vi "TDC_DAQV29_Paralled_muon.vi"(7 "address":string[](array[string])=["192.168.10.20"], 8 "error in (no error)":errorcluster, 9 "stop":bool, 10 "save data":bool=TRUE, 11 "SMA mode":bool) -> (0 "error out 3":errorcluster, 2 "csv path":path=path "D:/tdc/2017/data/test_20250311_101020.csv", 3 "rate":dbl=1.0823196338413628)   [LabVIEW 2017]
uses:
  gloabal.vi
  <vilib>/Utility/file.llb/Write Delimited Spreadsheet (DBL).vi
  <vilib>/Utility/file.llb/Write Delimited Spreadsheet (I64).vi
panel:
  out "pmt trigger rate":u32[](array[numeric])=[0, 35, 51, 19, 33, 19, 2704, 0, 64, 55, 26, 21, 70, 31, 43, 33, 76, 251, 28, 323, 16, 59, 106, 98, 0, 13, 2, 0, 53, 3, 0, 21, 65, 24, 240, 3, 89, 7, 48, 4, 0, 1, 60, 40, 0, 96, 100, 5, 11, 3, 0, 0, 0, 0, 0, 0, 0, 0, 0, 0, 0, 0, 0, 0]
  out "trigger rate":u64 format="%x"
  out "event":u32[](array[numeric])=[0, 0, 169, 166, 205, 191, 115, 111, 155, 143, 118, 110, 11836, 10970, 0, 0, 225, 211, 261, 248, 128, 116, 109, 106, 298, 278, 156, 146, 231, 218, 149, 126, 334, 315, 1087, 1060, 180, 172, 1669, 1652, 100, 96, 371, 351, 355, 349, 389, 370, 1, 1, 62, 58, 6, 6, 0, 0, 259, 253, 9, 8, 0, 0, 106, 100, 234, 213, 109, 106, 1110, 1086, 10, 9, 391, 374, 24, 24, 280, 267, 12, 12, 0, 0, 2, 2, 293, 271, 143, 136, 3, 3, 279, 187, 492, 458, 14, 13, 37, 35, 9, 8, 0, 0, 0, 0, 0, 0, 0, 0, 0, 0, 0, 0, 0, 0, 0, 0, 0, 0, 0, 0, 0, 0, 0, 0, 0, 0, 0, 0]
  in  "calib_file":path=path "D:/tdc/2017/data/test_20250311_110721_codeDensity.csv" caption="文件路径 （空时为对话框）"
  in  "use_calib_file":bool=TRUE
  out "cal 3":u32[](graph)=[0, 0, 0, 0, 0, 0, 0, 0, 0, 0, 0, 0, 0, 0, 0, 0, 0, 0, 0, 0, 0, 0, 0, 0, 0, 0, 0, 0, 0, 0, 0, 0, 0, 0, 0, 0, 0, 0, 0, 0, 0, 0, 0, 0, 0, 0, 0, 0, 0, 0, 0, 0, 0, 0, 0, 0, 0, 0, 0, 0, 0, 0, 0, 0, 0, 0, 0, 0, 0, 0, 0, 0, 0, 0, 0, 0, 0, 0, 0, 0, 0, 0, 0, 0, 0, 0, 0, 0, 0, 0, 0, 0, 0, 0, 0, 0, 0, 0, 0, 0, 0, 0, 0, 0, 0, 0, 0, 0, 0, 0, 0, 0, 0, 0, 0, 0, 0, 0, 0, 0, 0, 0, 0, 0, 0, 0, 0, 0, 0, 0, 0, 0, 0, 0, 0, 0, 0, 0, 0, 0, 0, 0, 0, 0, 0, 0, 0, 0, 0, 0, 0, 0, 0, 0, 0, 0, 0, 0, 0, 0, 0, 0, 0, 0, 0, 15, 3, 1, 14, 3, 31, 20, 16, 6, 1, 18, 12, 4, 29, 10, 8, 29, 2, 14, 4, 25, 7, 24, 4, 0, 1, 5, 8, 18, 22, 0, 4, 5, 0, 12, 9, 9, 20, 21, 4, 10, 13, 5, 21, 13, 14, 2, 6, 13, 1, 3, 5, 10, 20, 2, 3, 4, 3, 4, 2, 20, 13, 2, 5, 1, 3, 12, 4, 1, 14, 7, 5, 4, 1, 10, 2, 21, 14, 2, 5, 10, 4, 0, 11, 19, 6, 4, 1, 37, 1, 4, 2, 1, 10, 13, 4, 8, 10, 6, 9, 2, 0, 6, 8, 12, 3, 21, 5, 7, 8, 2, 3, 7, 17, 6, 5, 6, 4, 6, 0, 2, 1, 3, 10, 33, 7, 2, 6, 3, 7, 3, 2, 0, 12, 10, 11, 13, 13, 7, 3, 9, 6, 16, 0, 13, 5, 6, 3, 0, 5, 5, 7, 1, 10, 7, 13, 14, 5, 1, 12, 7, 1, 10, 2, 1, 14, 18, 13, 11, 4, 6, 9, 22, 11, 9, 2, 2, 8, 14, 4, 4, 6, 12, 13, 3, 9, 5, 5, 1, 5, 11, 18, 3, 0, 5, 4, 6, 7, 6, 1, 13, 5, 1, 2, 2, 1, 4, 12, 7, 3, 2, 3, 9, 11, 1, 20, 3, 4, 5, 5, 3, 5, 8, 5, 3, 26, 14, 6, 1, 3, 12, 12, 4, 23, 10, 3, 4, 4, 10, 3, 5, 4, 2, 14, 5, 15, 20, 1, 5, 1, 20, 6, 1, 3, 13, 21, 12, 7, 4, 1, 5, 30, 11, 2, 4, 0, 12, 7, 10, 3, 2, 25, 6, 1, 3, 6, 3, 8, 37, 4, 6, 2, 2, 4, 3, 5, 6, 13, 6, 9, 22, 1, 3, 7, 7, 4, 8, 33, 2, 1, 15, 3, 8, 23, 21, 2, 2, 27, 13, 3, 5, 10, 4, 18, 5, 5, 8, 0, 1, 8, 12, 4, 3, 0, 4, 8, 4, 7, 4, 2, 11, 13, 3, 0, 7, 5, 3, 4, 8, 4, 20, 2, 13, 4, 8, 6, 17, 4, 2, 1, 15, 2, 15, 5, 19, 0, 4, 15, 4, 16, 11, 1, 16, 4, 6, 6, 5, 7, 3, 9, 15, 3, 6, 3, 13, 5, 7, 3, 27, 2, 0, 21, 1, 4, 1, 4, 5, 3, 10, 7, 3, 6, 4, 18, 21, 7, 6, 7, 7, 12, 6, 9, 8, 11, 12, 13, 2, 2, 5, 4, 7, 52, 3, 5, 8, 7, 10, 4, 4, 6, 5, 18, 0, 3, 6, 1, 9, 5, 19, 13, 24, 12, 4, 4, 15, 6, 41, 3, 8, 5, 17, 26, 8, 7, 20, 2, 5, 12, 10, 10, 12, 9, 17, 6, 3, 1, 5, 3, 7, 8, 4, 10, 5, 10, 7, 1, 2, 14, 7, 25, 3, 0, 0, 0, 5, 21, 8, 14, 4, 10, 2, 3, 2, 4, 8, 12, 3, 6, 8, 3, 4, 3, 20, 5, 6, 7, 8, 11, 2, 8, 6, 5, 15, 17, 10, 10, 3, 3, 9, 18, 7, 7, 3, 5, 5, 5, 2, 2, 2, 4, 1, 0, 42, 3, 14, 4, 3, 5, 2, 7, 4, 2, 7, 5, 22, 4, 3, 17, 3, 5, 8, 19, 7, 5, 0, 3, 4, 10, 1, 8, 2, 2, 13, 23, 4, 9, 5, 0, 0, 0, 27, 2, 16, 11, 15, 3, 0, 18, 2, 8, 29, 19, 6, 7, 2, 6, 12, 1, 13, 2, 7, 5, 11, 8, 5, 6, 6, 19, 2, 4, 0, 7, 22, 13, 3, 7, 3, 8, 11, 0, 3, 26, 6, 5, 5, 6, 4, 10, 17, 16, 4, 3, 4, 3, 4, 21, 8, 10, 10, 7, 0, 9, 9, 2, 10, 10, 2, 9, 9, 4, 14, 5, 5, 4, 18, 6, 3, 0, 4, 1, 20, 2, 33, 4, 1, 2, 1, 20, 6, 3, 11, 10, 2, 1, 13, 9, 6, 1, 0, 0, 0, 0, 0, 0, 0, 0, 0, 0, 0, 0, 0, 0, 0, 0, 0, 0, 0, 0, 0, 0, 0, 0, 0, 0, 0, 0, 0, 0, 0, 0, 0, 0, 0, 0, 0, 0, 0, 0, 0, 0, 0, 0, 0, 0, 0, 0, 0, 0, 0, 0, 0, 0, 0, 0, 0, 0, 0, 0, 0, 0, 0, 0, 0, 0, 0, 0, 0, 0, 0, 0, 0, 0, 0, 0, 0, 0, 0, 0, 0, 0, 0, 0, 0, 0, 0, 0, 0, 0, 0, 0, 0, 0, 0, 0, 0, 0, 0, 0, 0, 0, 0, 0, 0, 0, 0, 0, 0, 0, 0, 0, 0, 0, 0, 0, 0, 0, 0, 0, 0, 0, 0, 0, 0, 0, 0, 0, 0, 0, 0, 0, 0, 0, 0, 0, 0, 0, 0, 0, 0, 0, 0, 0, 0, 0, 0, 0, 0, 0, 0, 0, 0, 0, 0, 0, 0, 0, 0, 0, 0, 0, 0, 0, 0, 0, 0, 0, 0, 0, 0, 0, 0, 0, 0, 0, 0, 0, 0, 0, 0, 0, 0, 0, 0, 0, 0, 0, 0, 0, 0, 0, 0, 0, 0, 0, 0, 0, 0, 0, 0, 0, 0, 0, 0, 0, 0, 0, 0, 0, 0, 0, 0, 0, 0, 0, 0, 0, 0, 0, 0, 0, 0, 0, 0, 0, 0, 0, 0, 0, 0, 0, 0, 0, 0, 0, 0, 0, 0, 0, 0, 0, 0, 0, 0, 0, 0, 0, 0, 0, 0, 0, 0, 0, 0, 0, 0, 0, 0, 0, 0, 0, 0, 0, 0, 0, 0, 0, 0, 0, 0, 0, 0, 0, 0, 0, 0, 0, 0, 0, 0, 0, 0, 0, 0, 0, 0, 0, 0, 0, 0, 0, 0, 0, 0, 0, 0, 0, 0, 0, 0, 0, 0, 0, 0, 0, 0, 0, 0, 0, 0, 0, 0, 0, 0, 0, 0, 0, 0, 0, 0, 0, 0, 0, 0, 0, 0, 0, 0, 0, 0, 0, 0, 0, 0, 0, 0, 0, 0, 0, 0, 0, 0, 0, 0, 0, 0, 0, 0, 0, 0, 0, 0, 0, 0, 0, 0, 0, 0, 0, 0, 0, 0, 0, 0, 0, 0, 0, 0, 0, 0, 0, 0, 0, 0, 0, 0, 0, 0, 0, 0, 0, 0, 0, 0, 0, 0, 0, 0, 0, 0, 0, 0, 0, 0, 0, 0, 0, 0, 0, 0, 0, 0, 0, 0, 0, 0, 0, 0, 0, 0, 0, 0, 0, 0, 0, 0, 0, 0, 0, 0, 0, 0, 0, 0, 0, 0, 0, 0, 0, 0, 0, 0, 0, 0, 0, 0, 0, 0, 0, 0, 0, 0, 0, 0, 0, 0, 0, 0, 0, 0, 0, 0, 0, 0, 0, 0, 0, 0, 0, 0, 0, 0, 0, 0, 0, 0, 0, 0, 0, 0, 0, 0, 0, 0, 0, 0, 0, 0, 0, 0, 0, 0, 0, 0, 0, 0, 0, 0, 0, 0, 0, 0, 0, 0, 0, 0, 0, 0, 0, 0, 0, 0, 0, 0, 0, 0, 0, 0, 0, 0, 0, 0, 0, 0, 0, 0, 0, 0, 0, 0, 0, 0, 0, 0, 0, 0, 0, 0, 0, 0, 0, 0, 0, 0, 0, 0, 0, 0, 0, 0, 0, 0, 0, 0, 0, 0, 0, 0, 0, 0, 0, 0, 0, 0, 0, 0, 0, 0, 0, 0, 0, 0, 0, 0, 0, 0, 0, 0, 0, 0, 0, 0, 0, 0, 0, 0, 0, 0, 0, 0, 0, 0, 0, 0, 0, 0, 0, 0, 0, 0, 0, 0, 0, 0, 0, 0, 0, 0, 0, 0, 0, 0, 0, 0, 0, 0, 0, 0, 0, 0, 0, 0, 0, 0, 0, 0, 0, 0, 0, 0, 0, 0, 0, 0, 0, 0, 0, 0, 0, 0, 0, 0, 0, 0, 0, 0, 0, 0, 0, 0, 0, 0, 0, 0, 0, 0, 0, 0, 0, 0, 0, 0, 0, 0, 0, 0, 0, 0, 0, 0, 0, 0, 0, 0, 0, 0, 0, 0, 0, 0, 0, 0, 0, 0, 0, 0, 0, 0, 0, 0, 0, 0, 0, 0, 0, 0, 0, 0, 0, 0, 0, 0, 0, 0, 0, 0, 0, 0, 0, 0, 0, 0, 0, 0, 0, 0, 0, 0, 0, 0, 0, 0, 0, 0, 0, 0, 0, 0, 0, 0, 0, 0, 0, 0, 0, 0, 0, 0, 0, 0, 0, 0, 0, 0, 0, 0, 0, 0, 0, 0, 0, 0, 0, 0, 0, 0, 0, 0, 0, 0, 0, 0, 0, 0, 0, 0, 0, 0, 0, 0, 0, 0, 0, 0, 0, 0, 0, 0, 0, 0, 0, 0, 0, 0, 0, 0, 0, 0, 0, 0, 0, 0, 0, 0, 0, 0, 0, 0, 0, 0, 0, 0, 0, 0, 0, 0, 0, 0, 0, 0, 0, 0, 0, 0, 0, 0, 0, 0, 0, 0, 0, 0, 0, 0, 0, 0, 0, 0, 0, 0, 0, 0, 0, 0, 0, 0, 0, 0, 0, 0, 0, 0, 0, 0, 0, 0, 0, 0, 0, 0, 0, 0, 0, 0, 0, 0, 0, 0, 0, 0, 0, 0, 0, 0, 0, 0, 0, 0, 0, 0, 0, 0, 0, 0, 0, 0, 0, 0, 0, 0, 0, 0, 0, 0, 0, 0, 0, 0, 0, 0, 0, 0, 0, 0, 0, 0, 0, 0, 0, 0, 0, 0, 0, 0, 0, 0, 0, 0, 0, 0, 0, 0, 0, 0, 0, 0, 0, 0, 0, 0, 0, 0, 0, 0, 0, 0, 0, 0, 0, 0, 0, 0, 0, 0, 0, 0, 0, 0, 0, 0, 0, 0, 0, 0, 0, 0, 0, 0, 0, 0, 0, 0, 0, 0, 0, 0, 0, 0, 0, 0, 0, 0, 0, 0, 0, 0, 0, 0, 0, 0, 0, 0, 0, 0, 0, 0, 0, 0, 0, 0, 0, 0, 0, 0, 0, 0, 0, 0, 0, 0, 0, 0, 0, 0, 0, 0, 0, 0, 0, 0, 0, 0, 0, 0, 0, 0, 0, 0, 0, 0, 0, 0, 0, 0, 0, 0, 0, 0, 0, 0, 0, 0, 0, 0, 0, 0, 0, 0, 0, 0, 0, 0, 0, 0, 0, 0, 0, 0, 0, 0, 0, 0, 0, 0, 0, 0, 0, 0, 0, 0, 0, 0, 0, 0, 0, 0, 0, 0, 0, 0, 0, 0, 0, 0, 0, 0, 0, 0, 0, 0, 0, 0, 0, 0, 0, 0, 0, 0, 0, 0, 0, 0, 0, 0, 0, 0, 0, 0, 0, 0, 0, 0, 0, 0, 0, 0, 0, 0, 0, 0, 0, 0, 0, 0, 0, 0, 0, 0, 0, 0, 0, 0, 0, 0, 0, 0, 0, 0, 0, 0, 0, 0, 0, 0, 0, 0, 0, 0, 0, 0, 0, 0, 0, 0, 0, 0, 0, 0, 0, 0, 0, 0, 0, 0, 0, 0, 0, 0, 0, 0, 0, 0, 0, 0, 0, 0, 0, 0, 0, 0, 0, 0, 0, 0, 0, 0, 0, 0, 0, 0, 0, 0, 0, 0, 0, 0, 0, 0, 0, 0, 0, 0, 0, 0, 0, 0, 0, 0, 0, 0, 0, 0, 0, 0, 0, 0, 0, 0, 0, 0, 0, 0, 0, 0, 0, 0, 0, 0, 0, 0, 0, 0, 0, 0, 0, 0, 0, 0, 0, 0, 0, 0, 0, 0, 0, 0, 0, 0, 0, 0, 0, 0, 0, 0]
  out "x+y":u64
  in  "coarse counter width":u16(ring) items=["29", "48"]
  out "name (unnamed)":string
  out "error out 5":errorcluster
  in  "timeout":dbl=30000.0
  out "DAC":dbl=8094.0
  out "Out":u8=3 format="%.0x"
  out "fine 4":u64=678912 format="%x"
  out "fine 3":u64=2652 format="%x"
  out "substring 3":string
  out "fine 2":u64=663 format="%x"
  out "substring 2":string
  out "substring":string
  in  "gps":bool
  out "Year":string="2025"
  in  "factor":i32=128
  in  "displayCR":bool=TRUE
  in  "Counter Setting":dbl=100000.0 format="%#_13g"
  in  "replace dat":bool
  in  "append csv":bool=TRUE
  out "element":string
  out "fine":u64=730 format="%x"
  in  "UDP Config":bool=TRUE
  in  "data  path":path=path "D:/tdc/2017/data"
  out "cal 2":u64[](graph)
  in  "Thresholds (mV)":dbl[](array[numeric])=[580.0, 580.0, 580.0, 580.0, 600.0, 600.0, 600.0, 600.0, 580.0, 580.0, 600.0, 600.0, 600.0, 600.0, 600.0, 600.0, 580.0, 580.0, 600.0, 600.0, 600.0, 600.0, 600.0, 600.0, 580.0, 580.0, 600.0, 600.0, 600.0, 600.0, 600.0, 600.0, 600.0, 600.0, 600.0, 600.0, 600.0, 600.0, 600.0, 600.0, 600.0, 600.0, 600.0, 600.0, 600.0, 600.0, 600.0, 600.0, 600.0, 600.0, 600.0, 600.0, 600.0, 600.0, 600.0, 600.0, 600.0, 600.0, 600.0, 600.0, 600.0, 600.0, 600.0, 600.0]
  out "error out 2":errorcluster
  in  "display":bool=TRUE
  in  "Thresholds":dbl=-0.03
  in  "one key for threshold":bool=TRUE
  in  "RST":bool
  in  "通道数量":i32=128
  out "Cal Table":u32[](array[numeric])=[100002, 100002, 100002, 100002, 100002, 100002, 100002, 100002, 100002, 100002, 100002, 100002, 100002, 100002, 100002, 100002, 100002, 100002, 100002, 100002, 100002, 100002, 100002, 100002, 100002, 100002, 100002, 100002, 100002, 100002, 100002, 100002, 100002, 100002, 100002, 100002, 100002, 100002, 100002, 100002, 100002, 100002, 100002, 100002, 100002, 100002, 100002, 100002, 100002, 100002, 100002, 100002, 100002, 100002, 100002, 100002, 100002, 100002, 100002, 100002, 100002, 100002, 100002, 100002, 100002, 100002, 100002, 100002, 100002, 100002, 100002, 100002, 100002, 100002, 100002, 100002, 100002, 100002, 100002, 100002, 100002, 100002, 100002, 100002, 100002, 100002, 100002, 100002, 100002, 100002, 100002, 100002, 100002, 100002, 100002, 100002, 100002, 100002, 100002, 100002, 100002, 100002, 100002, 100002, 100002, 100002, 100002, 100002, 100002, 100002, 100002, 100002, 100002, 100002, 100002, 100002, 100002, 100002, 100002, 100002, 100002, 100002, 100002, 100002, 100002, 100002, 100002, 100002]
  in  "channel for cal":i32=3
  out "channel number":u64=39
  out "Calibration Counter":i32=100000
  out "Event index":i32=97959
  out "cal":i64[](graph)=[0, 0, 0, 0, 0, 0, 0, 0, 0, 0, 0, 0, 0, 0, 0, 0, 0, 0, 0, 0, 0, 0, 0, 0, 0, 0, 0, 0, 0, 0, 0, 0, 0, 0, 0, 0, 0, 0, 0, 0, 0, 0, 0, 0, 0, 0, 0, 0, 0, 0, 0, 0, 0, 0, 0, 0, 0, 0, 0, 0, 0, 0, 0, 0, 0, 0, 0, 0, 0, 0, 0, 0, 0, 0, 0, 0, 0, 0, 0, 0, 0, 0, 0, 0, 0, 0, 0, 0, 0, 0, 0, 0, 0, 0, 0, 0, 0, 0, 0, 0, 0, 0, 0, 0, 0, 0, 0, 0, 0, 0, 0, 0, 0, 0, 0, 0, 0, 0, 0, 0, 0, 0, 0, 0, 0, 0, 0, 0, 0, 0, 0, 0, 0, 0, 0, 0, 0, 0, 0, 0, 0, 0, 0, 0, 0, 0, 0, 0, 0, 0, 0, 0, 0, 0, 0, 0, 0, 0, 0, 0, 0, 0, 0, 0, 0, 0, 0, 0, 39, 216, 172, 142, 327, 350, 408, 302, 198, 167, 268, 194, 181, 60, 483, 183, 195, 34, 304, 630, 47, 62, 33, 136, 75, 150, 139, 258, 262, 304, 39, 20, 34, 21, 32, 251, 47, 48, 349, 149, 273, 160, 100, 139, 241, 306, 184, 134, 88, 230, 233, 354, 57, 179, 31, 181, 100, 260, 286, 59, 137, 53, 165, 62, 108, 126, 103, 242, 183, 64, 58, 160, 293, 95, 287, 319, 129, 79, 261, 63, 352, 83, 224, 63, 79, 63, 383, 40, 33, 35, 298, 63, 190, 224, 201, 52, 128, 41, 46, 256, 165, 49, 169, 64, 44, 51, 216, 144, 100, 106, 448, 91, 109, 124, 62, 206, 35, 30, 379, 40, 42, 285, 34, 182, 58, 336, 295, 78, 260, 88, 52, 49, 336, 51, 140, 70, 284, 136, 48, 170, 42, 118, 255, 298, 31, 31, 17, 235, 135, 52, 156, 276, 145, 110, 67, 85, 35, 60, 49, 160, 53, 326, 410, 66, 98, 116, 75, 29, 20, 241, 80, 64, 342, 355, 132, 319, 65, 175, 40, 43, 801, 47, 156, 61, 223, 36, 41, 116, 747, 103, 37, 43, 103, 209, 119, 139, 344, 83, 89, 268, 89, 50, 28, 46, 42, 64, 163, 421, 143, 107, 35, 21, 63, 181, 231, 237, 243, 104, 86, 163, 145, 75, 112, 86, 52, 88, 294, 287, 49, 52, 70, 127, 60, 51, 218, 34, 83, 67, 525, 51, 52, 68, 101, 301, 164, 169, 166, 365, 50, 196, 44, 74, 101, 190, 128, 273, 138, 45, 215, 415, 57, 107, 307, 91, 210, 328, 40, 130, 48, 35, 15, 40, 136, 131, 187, 272, 64, 55, 67, 171, 190, 36, 31, 51, 93, 219, 51, 40, 466, 48, 32, 50, 417, 71, 45, 131, 116, 103, 59, 476, 103, 200, 157, 138, 60, 134, 194, 443, 94, 436, 67, 39, 62, 252, 40, 40, 81, 106, 68, 386, 229, 185, 91, 81, 160, 132, 192, 118, 48, 39, 119, 167, 185, 232, 106, 79, 61, 268, 91, 112, 112, 353, 161, 36, 32, 290, 182, 39, 82, 56, 91, 250, 43, 46, 77, 344, 81, 39, 336, 359, 42, 55, 100, 58, 80, 567, 92, 39, 79, 81, 263, 51, 109, 114, 358, 244, 70, 131, 116, 68, 54, 171, 344, 37, 105, 41, 32, 43, 481, 104, 368, 47, 142, 168, 95, 65, 18, 58, 83, 512, 53, 126, 181, 103, 58, 78, 217, 178, 64, 179, 301, 129, 350, 60, 74, 191, 196, 60, 70, 101, 54, 530, 117, 380, 54, 205, 95, 116, 106, 85, 107, 390, 47, 287, 48, 93, 87, 569, 368, 77, 128, 114, 748, 58, 130, 467, 60, 187, 224, 161, 138, 197, 150, 129, 101, 191, 247, 271, 49, 65, 248, 97, 39, 32, 297, 176, 173, 246, 165, 60, 39, 42, 86, 167, 812, 81, 59, 69, 54, 61, 47, 76, 139, 375, 53, 57, 137, 196, 98, 59, 51, 338, 202, 65, 85, 263, 49, 70, 42, 48, 478, 146, 73, 30, 43, 311, 224, 43, 398, 59, 72, 59, 84, 140, 65, 201, 232, 225, 40, 43, 117, 347, 40, 39, 99, 202, 210, 77, 238, 44, 48, 94, 222, 69, 54, 202, 113, 130, 55, 65, 246, 111, 51, 50, 310, 108, 124, 232, 43, 33, 34, 48, 450, 138, 133, 207, 53, 76, 199, 61, 137, 581, 57, 44, 179, 72, 216, 59, 482, 78, 63, 271, 86, 58, 75, 66, 59, 425, 49, 209, 218, 154, 57, 50, 79, 89, 176, 195, 271, 64, 24, 46, 378, 123, 452, 316, 33, 35, 235, 405, 56, 388, 81, 62, 58, 380, 351, 244, 51, 49, 37, 213, 158, 69, 481, 38, 31, 89, 84, 74, 199, 254, 339, 52, 115, 404, 46, 59, 156, 112, 65, 270, 48, 56, 233, 46, 177, 115, 100, 98, 259, 128, 126, 95, 49, 44, 342, 218, 47, 34, 35, 74, 215, 323, 113, 114, 298, 177, 242, 317, 63, 51, 243, 87, 97, 66, 4, 1, 0, 0, 0, 0, 0, 0, 0, 0, 0, 0, 0, 0, 0, 0, 0, 0, 0, 0, 0, 0, 0, 0, 0, 0, 0, 0, 0, 0, 0, 0, 0, 0, 0, 0, 0, 0, 0, 0, 0, 0, 0, 0, 0, 0, 0, 0, 0, 0, 0, 0, 0, 0, 0, 0, 0, 0, 0, 0, 0, 0, 0, 0, 0, 0, 0, 0, 0, 0, 0, 0, 0, 0, 0, 0, 0, 0, 0, 0, 0, 0, 0, 0, 0, 0, 0, 0, 0, 0, 0, 0, 0, 0, 0, 0, 0, 0, 0, 0, 0, 0, 0, 0, 0, 0, 0, 0, 0, 0, 0, 0, 0, 0, 0, 0, 0, 0, 0, 0, 0, 0, 0, 0, 0, 0, 0, 0, 0, 0, 0, 0, 0, 0, 0, 0, 0, 0, 0, 0, 0, 0, 0, 0, 0, 0, 0, 0, 0, 0, 0, 0, 0, 0, 0, 0, 0, 0, 0, 0, 0, 0, 0, 0, 0, 0, 0, 0, 0, 0, 0, 0, 0, 0, 0, 0, 0, 0, 0, 0, 0, 0, 0, 0, 0, 0, 0, 0, 0, 0, 0, 0, 0, 0, 0, 0, 0, 0, 0, 0, 0, 0, 0, 0, 0, 0, 0, 0, 0, 0, 0, 0, 0, 0, 0, 0, 0, 0, 0, 0, 0, 0, 0, 0, 0, 0, 0, 0, 0, 0, 0, 0, 0, 0, 0, 0, 0, 0, 0, 0, 0, 0, 0, 0, 0, 0, 0, 0, 0, 0, 0, 0, 0, 0, 0, 0, 0, 0, 0, 0, 0, 0, 0, 0, 0, 0, 0, 0, 0, 0, 0, 0, 0, 0, 0, 0, 0, 0, 0, 0, 0, 0, 0, 0, 0, 0, 0, 0, 0, 0, 0, 0, 0, 0, 0, 0, 0, 0, 0, 0, 0, 0, 0, 0, 0, 0, 0, 0, 0, 0, 0, 0, 0, 0, 0, 0, 0, 0, 0, 0, 0, 0, 0, 0, 0, 0, 0, 0, 0, 0, 0, 0, 0, 0, 0, 0, 0, 0, 0, 0, 0, 0, 0, 0, 0, 0, 0, 0, 0, 0, 0, 0, 0, 0, 0, 0, 0, 0, 0, 0, 0, 0, 0, 0, 0, 0, 0, 0, 0, 0, 0, 0, 0, 0, 0, 0, 0, 0, 0, 0, 0, 0, 0, 0, 0, 0, 0, 0, 0, 0, 0, 0, 0, 0, 0, 0, 0, 0, 0, 0, 0, 0, 0, 0, 0, 0, 0, 0, 0, 0, 0, 0, 0, 0, 0, 0, 0, 0, 0, 0, 0, 0, 0, 0, 0, 0, 0, 0, 0, 0, 0, 0, 0, 0, 0, 0, 0, 0, 0, 0, 0, 0, 0, 0, 0, 0, 0, 0, 0, 0, 0, 0, 0, 0, 0, 0, 0, 0, 0, 0, 0, 0, 0, 0, 0, 0, 0, 0, 0, 0, 0, 0, 0, 0, 0, 0, 0, 0, 0, 0, 0, 0, 0, 0, 0, 0, 0, 0, 0, 0, 0, 0, 0, 0, 0, 0, 0, 0, 0, 0, 0, 0, 0, 0, 0, 0, 0, 0, 0, 0, 0, 0, 0, 0, 0, 0, 0, 0, 0, 0, 0, 0, 0, 0, 0, 0, 0, 0, 0, 0, 0, 0, 0, 0, 0, 0, 0, 0, 0, 0, 0, 0, 0, 0, 0, 0, 0, 0, 0, 0, 0, 0, 0, 0, 0, 0, 0, 0, 0, 0, 0, 0, 0, 0, 0, 0, 0, 0, 0, 0, 0, 0, 0, 0, 0, 0, 0, 0, 0, 0, 0, 0, 0, 0, 0, 0, 0, 0, 0, 0, 0, 0, 0, 0, 0, 0, 0, 0, 0, 0, 0, 0, 0, 0, 0, 0, 0, 0, 0, 0, 0, 0, 0, 0, 0, 0, 0, 0, 0, 0, 0, 0, 0, 0, 0, 0, 0, 0, 0, 0, 0, 0, 0, 0, 0, 0, 0, 0, 0, 0, 0, 0, 0, 0, 0, 0, 0, 0, 0, 0, 0, 0, 0, 0, 0, 0, 0, 0, 0, 0, 0, 0, 0, 0, 0, 0, 0, 0, 0, 0, 0, 0, 0, 0, 0, 0, 0, 0, 0, 0, 0, 0, 0, 0, 0, 0, 0, 0, 0, 0, 0, 0, 0, 0, 0, 0, 0, 0, 0, 0, 0, 0, 0, 0, 0, 0, 0, 0, 0, 0, 0, 0, 0, 0, 0, 0, 0, 0, 0, 0, 0, 0, 0, 0, 0, 0, 0, 0, 0, 0, 0, 0, 0, 0, 0, 0, 0, 0, 0, 0, 0, 0, 0, 0, 0, 0, 0, 0, 0, 0, 0, 0, 0, 0, 0, 0, 0, 0, 0, 0, 0, 0, 0, 0, 0, 0, 0, 0, 0, 0, 0, 0, 0, 0, 0, 0, 0, 0, 0, 0, 0, 0, 0, 0, 0, 0, 0, 0, 0, 0, 0, 0, 0, 0, 0, 0, 0, 0, 0, 0, 0, 0, 0, 0, 0, 0, 0, 0, 0, 0, 0, 0, 0, 0, 0, 0, 0, 0, 0, 0, 0, 0, 0, 0, 0, 0, 0, 0, 0, 0, 0, 0, 0, 0, 0, 0, 0, 0, 0, 0, 0, 0, 0, 0, 0, 0, 0, 0, 0, 0, 0, 0, 0, 0, 0, 0, 0, 0, 0, 0, 0, 0, 0, 0, 0, 0, 0, 0, 0, 0, 0, 0, 0, 0, 0, 0, 0, 0, 0, 0, 0, 0, 0, 0, 0, 0, 0, 0, 0, 0, 0, 0, 0, 0, 0, 0, 0, 0, 0, 0, 0, 0, 0, 0, 0, 0, 0, 0, 0, 0, 0, 0, 0, 0, 0, 0, 0, 0, 0, 0, 0, 0, 0, 0, 0, 0, 0, 0, 0, 0, 0, 0, 0, 0, 0, 0, 0, 0, 0, 0, 0, 0, 0, 0, 0, 0, 0, 0, 0, 0, 0, 0, 0, 0, 0, 0, 0, 0, 0, 0, 0, 0, 0, 0, 0, 0, 0, 0, 0, 0, 0, 0, 0, 0, 0, 0, 0, 0, 0, 0, 0, 0, 0, 0, 0, 0, 0, 0, 0, 0, 0, 0, 0, 0, 0, 0, 0, 0, 0, 0, 0, 0, 0, 0, 0, 0, 0, 0, 0, 0, 0, 0, 0, 0, 0, 0, 0, 0, 0, 0, 0, 0, 0, 0, 0, 0, 0, 0, 0, 0, 0, 0, 0, 0, 0, 0, 0, 0, 0, 0, 0, 0, 0, 0, 0, 0, 0, 0, 0, 0, 0, 0, 0, 0, 0, 0, 0, 0, 0, 0, 0, 0, 0, 0, 0, 0, 0, 0, 0, 0, 0, 0, 0, 0, 0, 0, 0, 0, 0, 0, 0, 0, 0, 0, 0, 0, 0, 0, 0, 0, 0, 0, 0, 0, 0, 0, 0, 0, 0, 0, 0, 0, 0, 0, 0, 0, 0, 0, 0, 0, 0, 0, 0, 0, 0, 0, 0, 0, 0, 0, 0, 0, 0, 0, 0, 0, 0, 0, 0, 0, 0, 0, 0, 0, 0, 0, 0, 0, 0, 0, 0, 0, 0, 0, 0, 0, 0, 0, 0, 0, 0, 0, 0, 0, 0, 0, 0, 0, 0, 0, 0, 0, 0, 0, 0, 0, 0, 0, 0, 0, 0, 0, 0, 0, 0, 0, 0, 0, 0, 0, 0, 0, 0, 0, 0, 0, 0, 0, 0, 0, 0, 0, 0, 0, 0, 0, 0, 0, 0, 0, 0, 0, 0, 0, 0, 0, 0, 0, 0, 0, 0, 0, 0, 0]
  out "error out":errorcluster
  out "appended path":path=path "D:/tdc/2017/data/test_20250311_101020.dat"
  in  "filename":string="test"
  in  "Events":i32=110000 min=1
  in  "timeout (ms)":i32=10000
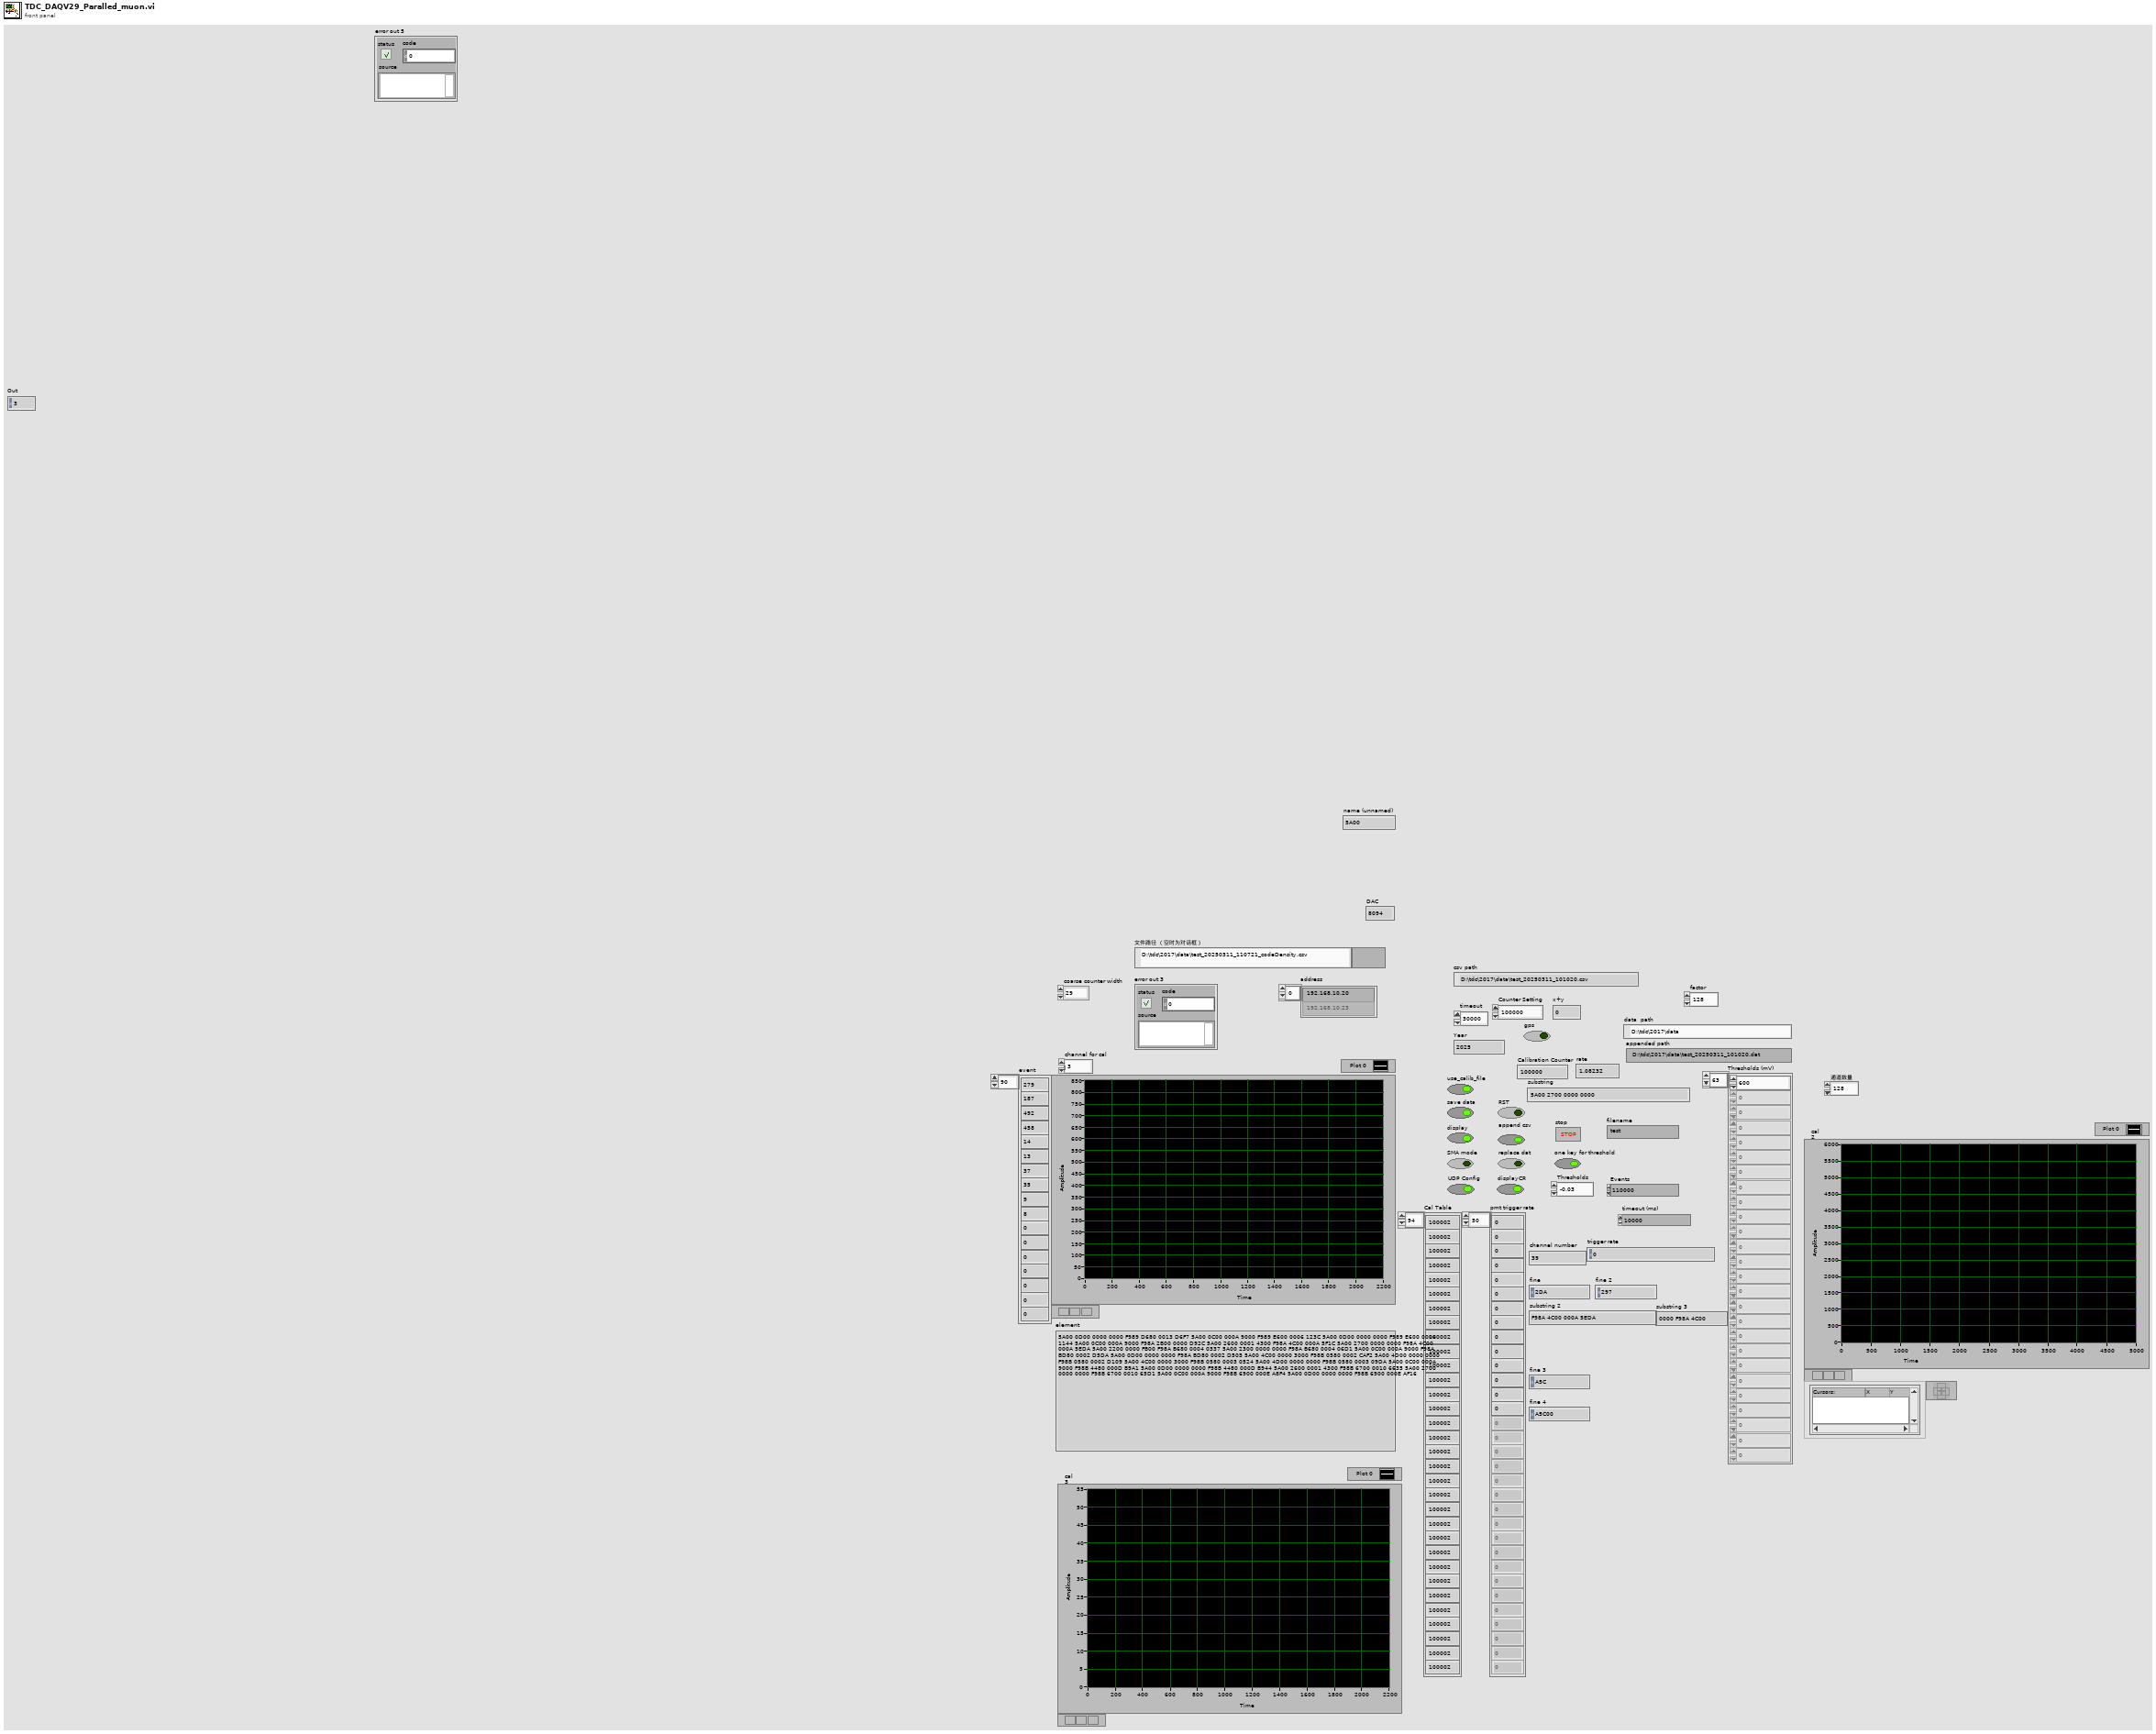
[diagram p1: front panel]
types:
  T1 = enum16{"open", "replace", "create", "open or create", "replace or create", "replace or create with confirmation"}
  T2 = enum16{"big-endian, network order", "native, host order", "little-endian"}
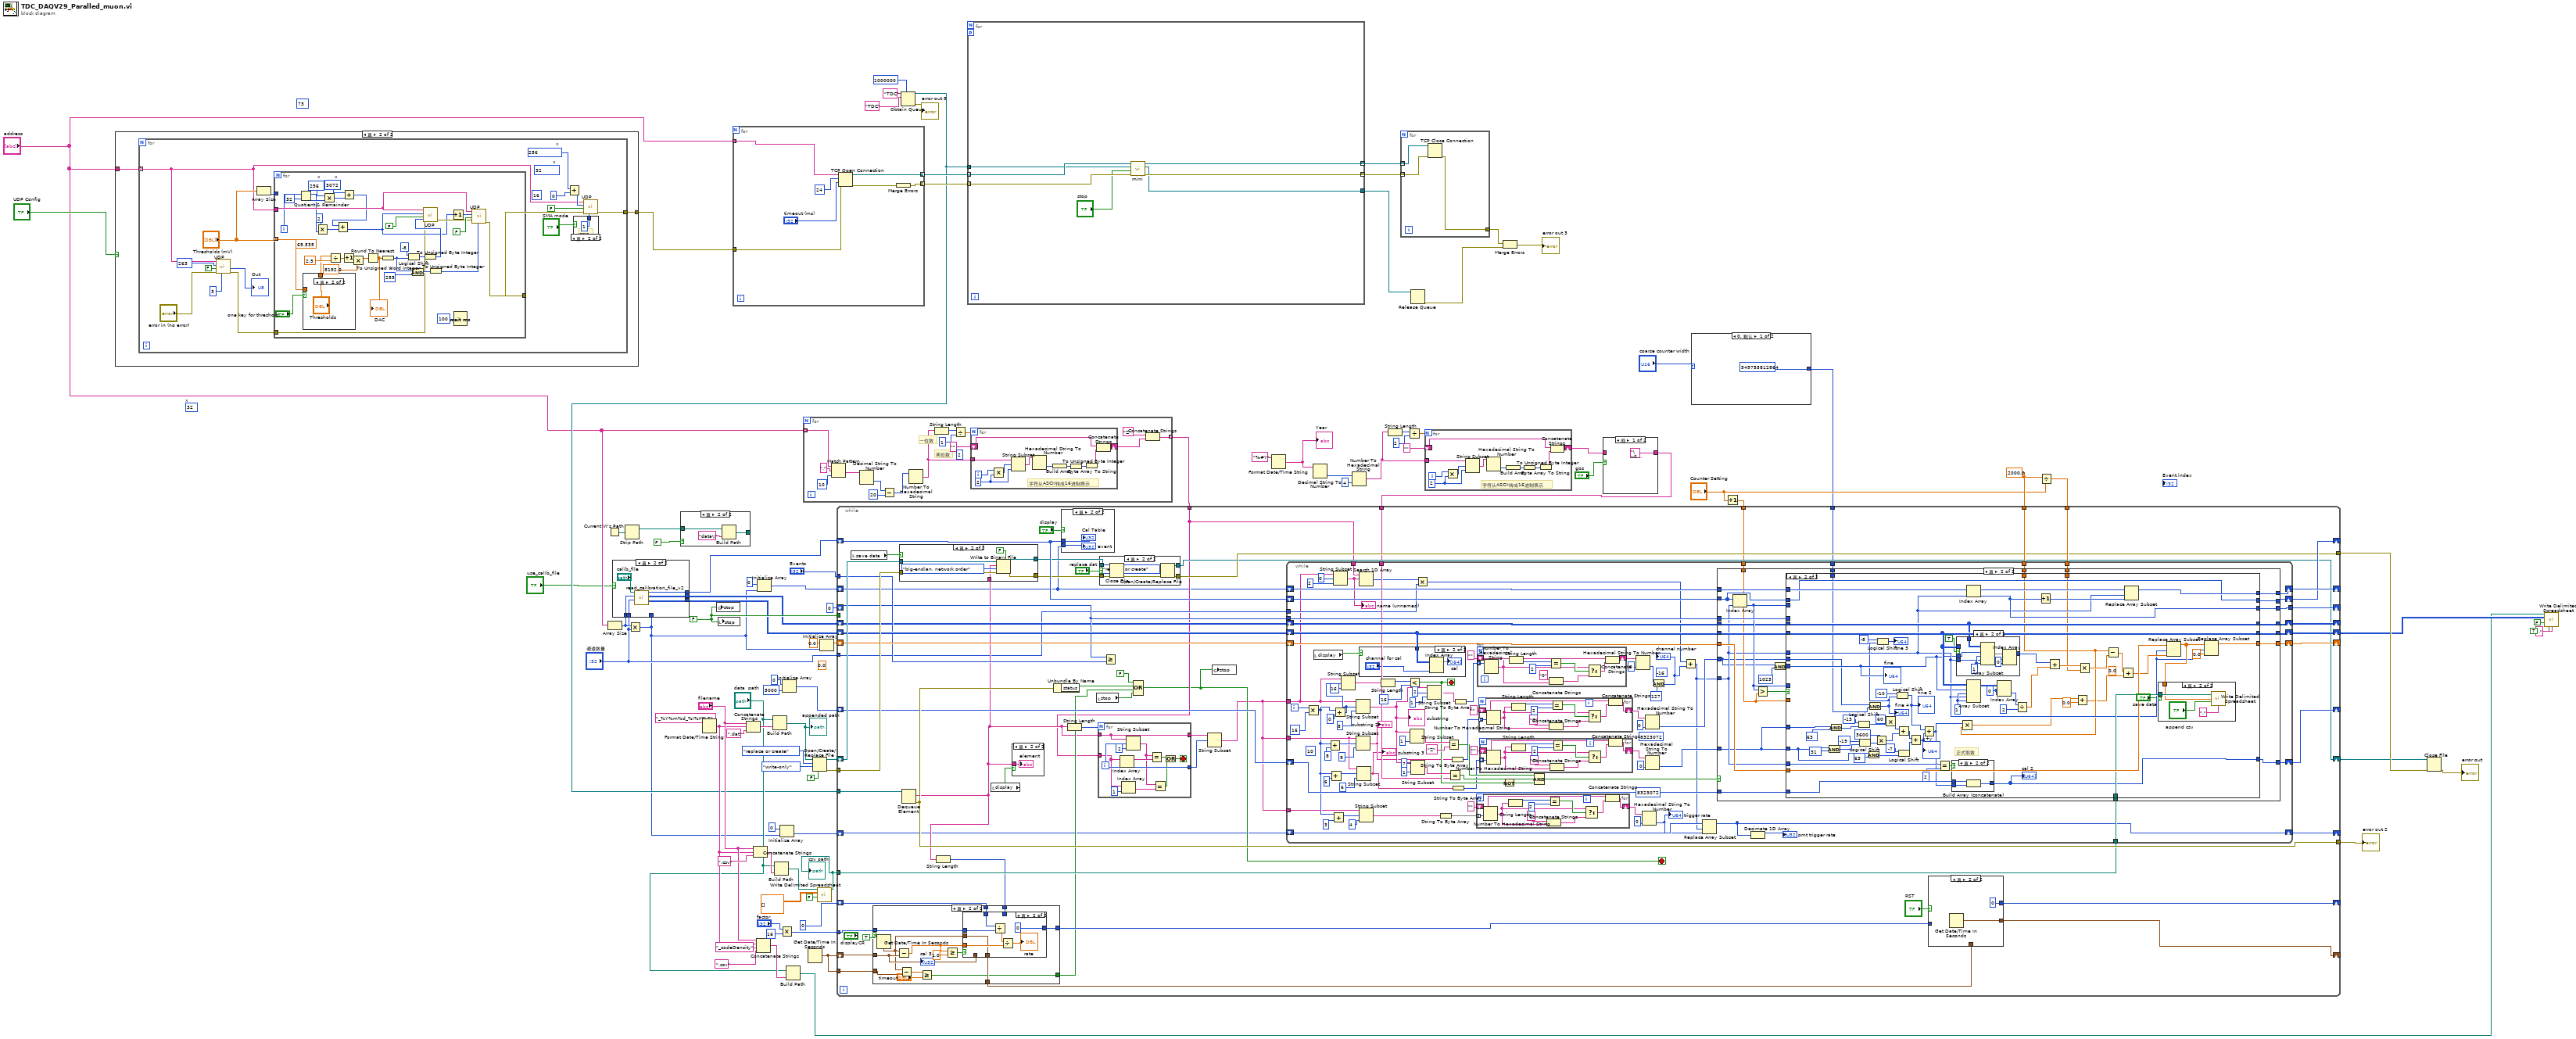
[diagram p0: block diagram]
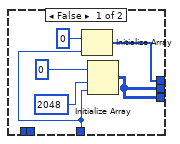
[diagram p2: hidden frame]
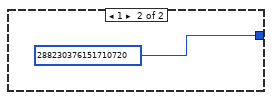
[diagram p3: hidden frame]
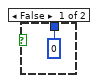
[diagram p6: hidden frame]
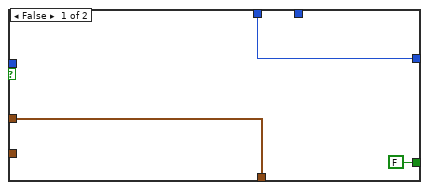
[diagram p12: hidden frame]
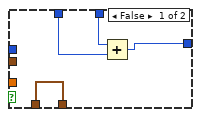
[diagram p13: hidden frame]
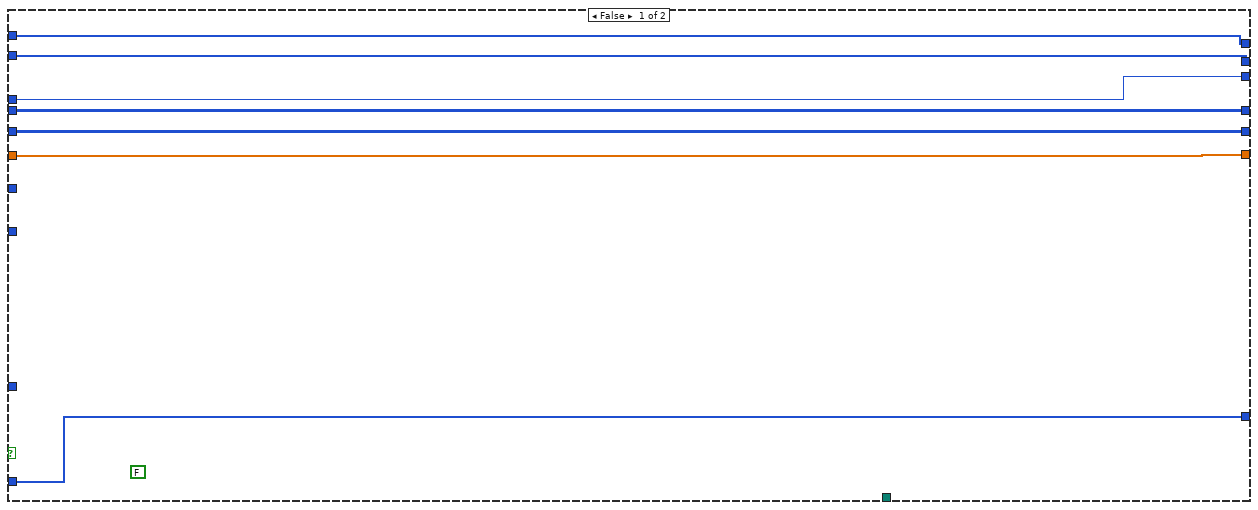
[diagram p17: hidden frame]
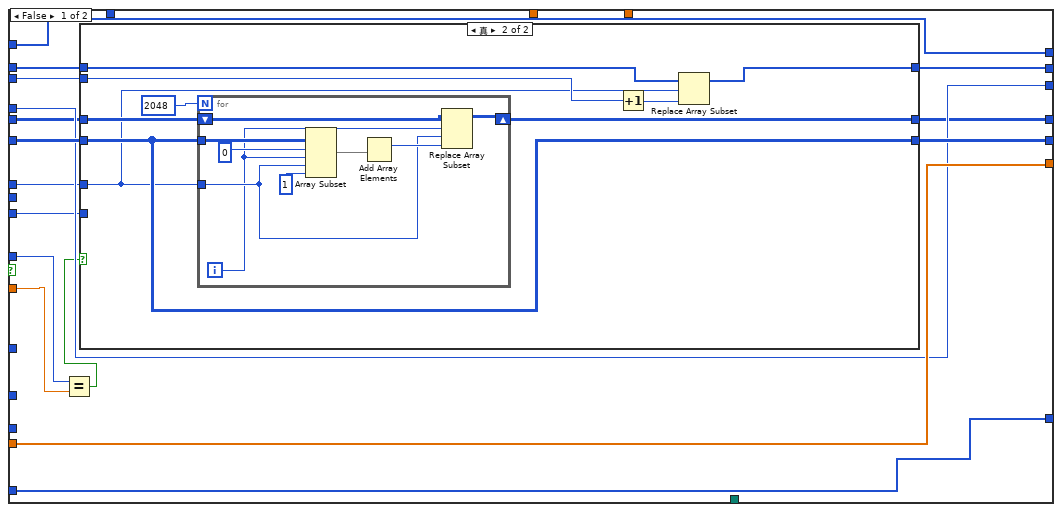
[diagram p18: hidden frame]
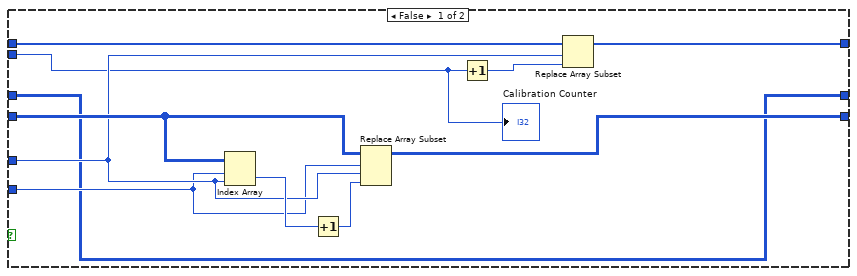
[diagram p19: hidden frame]
diagram:
  (unwired) u32 73 ("Address")
  w51 = 2000.0 ("x")
  (unwired) u16 32  # x
  w13 = FALSE ("stop")
  (unwired) 0.0
  n1 = case shown="真" "UDP Config" {
    tunnel: "address" -> [_ w93]
    tunnel: [_ w94] -> w18
    frame False {
    }
    frame True {
      n2 = for {
        tunnel: [w109] -> w94
        tunnel: w93 -> [w97] mode=indexing
        (unwired) u16 32  # x
        (unwired) u32 16 ("Address")
        w102 = u16 256  # x
        n3 = call "UDP.vi"("In"=u8 3, "error in (no error)"="error in (no error)", "Read (TRUE)"=FALSE, "Address"=u32 263, "IP address"=w97) -> ("error out"=w95:errorcluster, "Out"=→"Out":u8)  [unwired: 4 in]
        n4 = Array Size(array="Thresholds (mV)") -> (size(s)=w106:i32)
        n5 = for {
          tunnel: w97 -> [w143]
          tunnel: "Thresholds (mV)" -> [w130] mode=indexing
          tunnel: [w133] -> w110
          tunnel: w106 -> [_]
          tunnel: w95 -> [w117]
          i -> [w125]
          (unwired) 65.535 ("y")
          w126 = u16 3072  # x
          w127 = u16 256  # x
          w139 = u16 255  # x
          n6 = Quotient & Remainder(x=w125, y=32) -> (x-y*floor(x/y)=w119:i32, floor(x/y)=w128:i32)
          n7 = case shown="真" "one key for threshold" {
            tunnel: [w149 "Thresholds"] -> w131
            tunnel: w130 -> [w149 _]
            frame False {
            }
            frame True {
            }
          }
          n8 = Multiply(x=2, y=w119) -> (x*y=w120:i32)
          n9 = Multiply(x=w127, y=w128) -> (x*y=w122:i32)
          n10 = Divide(x=w131, y=2.5) -> (x/y=w146:dbl)
          n11 = Increment(x=w146) -> (x+1=w116:dbl)
          n12 = Add(x=w126, y=w122) -> (x+y=w121:i32)
          n13 = Add(x=w121, y=w120) -> (x+y=w124:i32)
          n14 = Multiply(x=w116, y=8192.0) -> (x*y=w115:dbl)
          n15 = Round To Nearest(number=w115) -> (nearest integer value=w144:dbl)
          "DAC" <- w144
          n16 = To Unsigned Word Integer(number=w144) -> (unsigned 16bit integer=w135:u16)
          n17 = Logical Shift(y=i16 -8, x=w135) -> (x << y=w141:u16)
          n18 = And(x=w135, y=w139) -> (x .and. y?=w138:u16)
          n19 = To Unsigned Byte Integer(number=w141) -> (unsigned 8bit integer=w140:u8)
          n20 = call "UDP.vi"("In"=w140, "error in (no error)"=w117, "Read (TRUE)"=FALSE, "Address"=w124, "IP address"=w143) -> ("error out"=w134:errorcluster)  [unwired: 4 in, 1 out]
          n21 = To Unsigned Byte Integer(number=w138) -> (unsigned 8bit integer=w137:u8)
          n22 = Increment(x=w124) -> (x+1=w123:i32)
          n23 = Wait (ms)(milliseconds to wait=u32 100) -> ()  [unwired: 1 out]
          n24 = call "UDP.vi"("In"=w137, "error in (no error)"=w134, "Read (TRUE)"=FALSE, "Address"=w123, "IP address"=w143) -> ("error out"=w133:errorcluster)  [unwired: 4 in, 1 out]
        }
        n25 = Add(x=w102, y=u32 0 ("Address")) -> (x+y=w103:u32)
        n26 = case shown="真" "SMA mode" {
          tunnel: [u8 0 ("In") u8 1 ("In")] -> w108
          frame False {
          }
          frame True {
            # "sma"
          }
        }
        n27 = call "UDP.vi"("In"=w108, "error in (no error)"=w110, "Read (TRUE)"=FALSE, "Address"=w103, "IP address"=w97) -> ("error out"=w109:errorcluster)  [unwired: 4 in, 1 out]
      }
    }
  }
  n28 = Current VI's Path() -> (path=w87:path)
  n29 = Array Size(array="address") -> (size(s)=w5:i32)
  n30 = Strip Path(path=w87) -> (stripped path=w86:path)  [unwired: 1 out]
  n31 = Multiply(x=w5, y="通道数量") -> (x*y=w2:i32)
  n32 = case shown="真" "use_calib_file" {
    tunnel: w2 -> [w154 _]
    tunnel: [w151 w162] -> w8
    tunnel: [w151 w161] -> w7
    tunnel: [w152 w160] -> w6
    tunnel: w5 -> [_ w159]
    tunnel: "通道数量" -> [_ w158]
    frame False {
      n33 = Initialize Array(u32 0 ("element"), w154) -> (w152:u32[])
      n34 = Initialize Array(u32 0 ("element"), 2048 ("dimension size"), w154) -> (w151:u32[][])
    }
    frame True {
      n35 = call "read_calibration_file_v2.vi"("通道数量"=w158, "板子数量"=w159, "file path (dialog if empty)"="calib_file") -> ("code_density"=w162:i64[][], "accumulation"=w161:u32[][], "Cal Table"=w160:u32[])  [unwired: 5 in, 1 out]
    }
  }
  n36 = case shown="真" FALSE {
    tunnel: w86 -> [w163 w165]
    tunnel: [w163 w164] -> _
    frame False {
    }
    frame True {
      n37 = Build Path(base path=w165, name or relative path="data\\") -> (appended path=w164:path)
    }
  }
  n38 = Format Date/Time String(time format string (%c)="_%Y%m%d_%I%M%S") -> (date/time string=w68:string)  [unwired: 2 in]
  n39 = global write "gloabal.vi" "stop"(w13) -> ()
  n40 = local write "stop"(w13) -> ()
  n41 = for {
    tunnel: "address" -> [w172] mode=indexing
    tunnel: [w171] -> w28 mode=indexing
    tunnel: [w169] -> w27 mode=indexing
    tunnel: w18 -> [w168]
    n42 = TCP Open Connection(address=w172, remote port or service name=u16 24 ("port"), timeout ms (60000)="timeout (ms)", error in (no error)=w168) -> (connection ID=w171:refnum<k5>, error out=w170:errorcluster)  [unwired: 1 in]
    n43 = Merge Errors(w170) -> (w169:errorcluster)
  }
  n44 = Concatenate Strings("filename", w68, ".dat") -> (w85:string)
  n45 = Concatenate Strings("filename", w68, ".csv") -> (w75:string)
  n46 = Concatenate Strings("filename", w68, "_codeDensity" ("string"), ".csv") -> (w65:string)
  n47 = Initialize Array(u32 0 ("element"), w2) -> (w74:u32[])
  n48 = Build Path(base path="data  path", name or relative path=w85) -> (appended path=w84:path)
  "appended path" <- w84
  n49 = Build Path(base path="data  path", name or relative path=w75) -> (appended path=w72:path)
  n50 = Initialize Array(u32 0 ("element"), w2) -> (w1:u32[])
  n51 = Multiply(x="factor", y=16) -> (x*y=w44:i32)
  n52 = Initialize Array(u32 0 ("element"), 5000 ("dimension size")) -> (w56:u32[])
  n53 = Build Path(base path="data  path", name or relative path=w65) -> (appended path=w62:path)
  n54 = for {
    tunnel: [w175] -> w30 mode=indexing
    tunnel: "address" -> [w174] mode=indexing
    (unwired) 2 ("y")
    # "一位数"
    # "两位数"
    n55 = Match Pattern(string=w174, regular expression="." ("search string"), offset (0)=10) -> (after substring=w181:string)  [unwired: 3 out]
    n56 = Decimal String To Number(string=w181) -> (number=w178:i32)  [unwired: 2 in, 1 out]
    n57 = Subtract(x=w178, y=20) -> (x-y=w177:i32)
    n58 = Number To Hexadecimal String(2:w177) -> (0:w180:string)  [unwired: 1 in]
    n59 = String Length(string=w180) -> (length=w186:i32)
    n60 = Divide(x=w186, y=1) -> (x/y=w187:dbl)
    n61 = for {
      N: w187 -> [_]
      shift-right: [w199] -> w176
      shift-left: "" ("format string") -> [w198]
      tunnel: w180 -> [w189]
      i -> [w197]
      w191 = 2 ("y")
      # "字符从ASCII转成16进制表示"
      n62 = Multiply(x=w197, y=w191) -> (x*y=w190:i32)
      n63 = String Subset(string=w189, offset (0)=w190, length (rest)=w191) -> (substring=w192:string)
      n64 = Hexadecimal String To Number(string=w192) -> (number=w196:u32)  [unwired: 2 in, 1 out]
      n65 = Build Array(w196) -> (w195:u32[])
      n66 = To Unsigned Byte Integer(number=w195) -> (unsigned 8bit integer=w194:u8[])
      n67 = Byte Array To String(unsigned byte array=w194) -> (string=w193:string)
      n68 = Concatenate Strings(w198, w193) -> (w199:string)
    }
    n69 = Concatenate Strings("Z", w176) -> (w175:string)
  }
  n70 = Get Date/Time In Seconds() -> (seconds since 1Jan1904=w29:timestamp)
  n71 = Open/Create/Replace File(file path (use dialog)=w84, operation (0:open)=T1."replace or create", access (0:read/write)=enum16{"read/write", "read-only", "write-only"}."write-only", disable buffering (F)=FALSE) -> (refnum out=w89:refnum<file>, error out=w88:errorcluster)  [unwired: 2 in, 1 out]
  n72 = call-poly <vilib>:"Write Delimited Spreadsheet.vi"("file path (dialog if empty)"=w72, "2D data"=dbl[][] [], "append to file? (new file:F)"=FALSE) -> ("new file path (Not A Path if cancelled)"=w12:path)  [unwired: 11 in, 1 out]
  "csv path" <- w12
  n73 = Initialize Array(0.0, w2) -> (w58:dbl[])
  n74 = Obtain Queue(max queue size (-1, unlimited)=1000000, name (unnamed)="TDC", element data type="TDC" ("name (unnamed)")) -> (queue out=w19:refnum<queue>, error out=→"error out 5":errorcluster)  [unwired: 2 in, 1 out]
  n75 = for {
    tunnel: w28 -> [w206] mode=indexing
    tunnel: w27 -> [w205] mode=indexing
    tunnel: [w204] -> w26 mode=indexing
    tunnel: [w203] -> w25 mode=indexing
    workers-P: _ -> [_]
    tunnel: w19 -> [w202]
    tunnel: [w201] -> w20
    n76 = call "mini.vi"("error in (no error)"=w205, "stop"="stop", "queue out 2"=w202, "connection ID 2"=w206) -> ("error out 3"=w203:errorcluster, "queue out"=w201:refnum<queue>, "connection ID"=w204:refnum<k5>)  [unwired: 5 in]
  }
  n77 = Format Date/Time String(time format string (%c)="%#Y") -> (date/time string=w41:string)  [unwired: 2 in]
  "Year" <- w41
  n78 = Decimal String To Number(string=w41) -> (number=w40:i32)  [unwired: 2 in, 1 out]
  n79 = Number To Hexadecimal String(1:i16 4 ("width (-)"), 2:w40) -> (0:w34:string)
  n80 = String Length(string=w34) -> (length=w36:i32)
  n81 = for {
    tunnel: w26 -> [w209] mode=indexing
    tunnel: w25 -> [w208] mode=indexing
    tunnel: [w207] -> w17
    n82 = TCP Close Connection(connection ID=w209, error in (no error)=w208) -> (error out=w207:errorcluster)  [unwired: 1 in, 1 out]
  }
  n83 = Divide(x=w36, y=2) -> (x/y=w37:dbl)
  n84 = Release Queue(queue=w20) -> (error out=w16:errorcluster)  [unwired: 2 in, 2 out]
  n85 = for {
    N: w37 -> [_]
    shift-right: [w220] -> w33
    shift-left: "" ("format string") -> [w219]
    tunnel: w34 -> [w210]
    i -> [w218]
    w212 = 2 ("y")
    # "字符从ASCII转成16进制表示"
    n86 = Multiply(x=w218, y=w212) -> (x*y=w211:i32)
    n87 = String Subset(string=w210, offset (0)=w211, length (rest)=w212) -> (substring=w213:string)
    n88 = Hexadecimal String To Number(string=w213) -> (number=w217:u32)  [unwired: 2 in, 1 out]
    n89 = Build Array(w217) -> (w216:u32[])
    n90 = To Unsigned Byte Integer(number=w216) -> (unsigned 8bit integer=w215:u8[])
    n91 = Byte Array To String(unsigned byte array=w215) -> (string=w214:string)
    n92 = Concatenate Strings(w219, w214) -> (w220:string)
  }
  n93 = Merge Errors(w17, w16) -> (→"error out 3":errorcluster)
  n94 = case shown="假" "gps" {
    tunnel: w33 -> [_ w222]
    tunnel: ["\u0000" ("format string") w222] -> w32
    frame False {
    }
    frame True {
    }
  }
  n95 = case shown="0, 默认" "coarse counter width" {
    tunnel: [u64 549755812864 ("port") u64 288230376151710720 ("port")] -> w10
    frame 0, Default {
    }
    frame 1 {
    }
  }
  n96 = Increment(x="Counter Setting") -> (x+1=w47:dbl)
  n97 = Divide(x=w51, y="Counter Setting") -> (x/y=w50:dbl)
  n98 = while {
    tunnel: w88 -> [w282]
    tunnel: [w262] -> w59
    tunnel: [w251] -> w81
    shift-right: [w279] -> w63
    shift-left: w8 -> [w280]
    shift-right: [w271] -> _
    shift-left: w58 -> [w278]
    tunnel: "Events" -> [w277]
    shift-right: [w276] -> _
    shift-left: w74 -> [w228]
    shift-right: [w275] -> _
    shift-left: u32 0 ("element") -> [w274]
    shift-right: [w273] -> _
    shift-left: w6 -> [w264]
    shift-right: [w266] -> _
    shift-left: w7 -> [w272]
    tunnel: w12 -> [w258]
    shift-right: [w270] -> _
    shift-left: 0 -> [w245]
    shift-right: [w268] -> _
    shift-left: w29 -> [w267]
    tunnel: w13 -> [_]
    tunnel: w19 -> [w263]
    shift-right: [w259] -> _
    shift-left: w56 -> [w260]
    tunnel: w30 -> [w232]
    tunnel: w51 -> [w256]
    tunnel: w50 -> [w255]
    shift-right: [w250] -> w49
    shift-left: w89 -> [w281]
    tunnel: w47 -> [w249]
    tunnel: w44 -> [w242]
    tunnel: w32 -> [w240]
    tunnel: w29 -> [w239]
    tunnel: "通道数量" -> [w233]
    tunnel: w10 -> [w229]
    shift-right: [w225] -> _
    shift-left: w1 -> [w226]
    stop <- w231 stop-if-true
    n99 = local read "save data"() -> (w244:bool)
    n100 = Dequeue Element(queue=w263) -> (element=w235:string, error out=w262:errorcluster)  [unwired: 2 in, 2 out]
    n101 = case shown="真" w244 {
      tunnel: w282 -> [w295 w303]
      tunnel: w281 -> [w296 w302]
      tunnel: w235 -> [_ w299]
      tunnel: [w296 w298] -> w254
      tunnel: [w295 w297] -> w252
      frame False {
      }
      frame True {
        n102 = Write to Binary File(file (use dialog)=w302, data=w299, error in=w303, 5:FALSE ("prepend array or string size? (T)"), 9:T2."big-endian, network order" ("byte order (0:big-endian, network order)")) -> (refnum out=w298:refnum<file>, error out=w297:errorcluster)  [unwired: 1 in, 1 out]
      }
    }
    n103 = String Length(string=w235) -> (length=w246:i32)
    n104 = case shown="真" TRUE {
      tunnel: w267 -> [w315 w325]
      tunnel: [w315 w326] -> w248
      tunnel: w245 -> [w314 w324]
      tunnel: w246 -> [_ w323]
      tunnel: [w314 w322] -> w247
      tunnel: w242 -> [_ w321]
      tunnel: w239 -> [_ w319]
      tunnel: [FALSE w316] -> w238
      frame False {
      }
      frame True {
        n105 = Get Date/Time In Seconds() -> (seconds since 1Jan1904=w320:timestamp)
        n106 = Subtract(x=w320, y=w325) -> (x-y=w328:dbl)
        n107 = Subtract(x=w320, y=w319) -> (x-y=w318:dbl)
        n108 = Greater Or Equal?(x=w318, y="timeout") -> (x >= y?=w316:bool)
        n109 = Greater Or Equal?(x=w328, y=1.0) -> (x >= y?=w329:bool)
        n110 = case shown="真" w329 {
          tunnel: w328 -> [_ w340]
          tunnel: w320 -> [_ w338]
          tunnel: [w333 w338] -> w326
          tunnel: w325 -> [w333 _]
          tunnel: w324 -> [w332 w335]
          tunnel: w323 -> [w331 _]
          tunnel: [w330 0] -> w322
          tunnel: w321 -> [_ w334]
          frame False {
            n111 = Add(x=w331, y=w332) -> (x+y=w330:i32)
          }
          frame True {
            n112 = Divide(x=w335, y=w334) -> (x/y=w337:dbl)
            n113 = Divide(x=w337, y=w340) -> (x/y=→"rate":dbl)
          }
        }
      }
    }
    n114 = local read "display"() -> (w243:bool)
    n115 = case shown="真" w243 {
      tunnel: w235 -> [_ w294]
      frame False {
      }
      frame True {
        "element" <- w294
      }
    }
    n116 = Unbundle By Name(w262) -> ("status"=w261:bool)
    n117 = case shown="真" "display" {
      tunnel: w264 -> [_ w342]
      tunnel: w228 -> [_ w341]
      frame False {
      }
      frame True {
        "Cal Table" <- w342
        "event" <- w341
      }
    }
    n118 = String Length(string=w235) -> (length=w237:i32)
    n119 = local read "stop"() -> (w230:bool)
    n120 = for {
      N: w237 -> [_]
      tunnel: w235 -> [w291]
      tunnel: [w291] -> w236
      tunnel: [w290] -> w234
      tunnel: w232 -> [w288]
      i -> [w290]
      stop <- w284 stop-if-true
      n121 = Index Array(array=w288) -> (element=w289:string)  [unwired: 1 in]
      n122 = Index Array(array=w288, index=1) -> (element=w286:string)
      n123 = String Subset(string=w291, offset (0)=w290, length (rest)=2 ("length (rest)")) -> (substring=w285:string)
      n124 = Equal?(x=w285, y=w289) -> (x = y?=w292:bool)
      n125 = Equal?(x=w285, y=w286) -> (x = y?=w283:bool)
      n126 = Or(x=w292, y=w283) -> (x .or. y?=w284:bool)
    }
    n127 = case shown="真" "replace dat" {
      tunnel: w254 -> [w305 w311]
      tunnel: [w305 w310] -> w250
      tunnel: w252 -> [w304 w307]
      tunnel: [w304 w306] -> w251
      frame False {
      }
      frame True {
        n128 = Close File(refnum=w311, error in=w307) -> (path=w312:path, error out=w308:errorcluster)
        n129 = Open/Create/Replace File(file path (use dialog)=w312, error in=w308, operation (0:open)=T1."replace or create") -> (refnum out=w310:refnum<file>, error out=w306:errorcluster)  [unwired: 3 in, 1 out]
      }
    }
    n130 = Greater Or Equal?(x=w274, y=w277) -> ()  [unwired: 1 out]
    n131 = Compound Arithmetic op=OR(FALSE ("x"), w261, w238, w230) -> (w231:bool)
    n132 = String Subset(string=w236, offset (0)=w234) -> (substring=w227:string)  [unwired: 1 in]
    n133 = global write "gloabal.vi" "stop"(w231) -> ()
    n134 = while {
      tunnel: w227 -> [w366]
      shift-right: [w436] -> w279
      shift-left: w280 -> [w434]
      shift-right: [w432] -> w271
      shift-left: w278 -> [w433]
      shift-right: [w429] -> w276
      shift-left: w228 -> [w428]
      tunnel: [w427] -> w275
      tunnel: w274 -> [w426]
      shift-right: [w424] -> w273
      shift-left: w264 -> [w425]
      tunnel: w258 -> [w422]
      shift-right: [w421] -> w266
      shift-left: w272 -> [w391]
      shift-right: [w418] -> w259
      shift-left: w260 -> [w419]
      tunnel: w227 -> [w385]
      tunnel: w256 -> [w398]
      tunnel: w255 -> [w397]
      tunnel: w249 -> [w390]
      tunnel: w240 -> [w380]
      tunnel: w233 -> [w368]
      tunnel: w232 -> [w367]
      tunnel: w229 -> [w363]
      tunnel: w227 -> [w352]
      shift-right: [w348] -> w225
      shift-left: w226 -> [w351]
      i -> [w437]
      stop <- w393 stop-if-true
      (unwired) u64 8323072 ("port")
      (unwired) 10 ("length (rest)")
      (unwired) u64 8323072 ("port")
      (unwired) i16 -16 ("y")
      n135 = Multiply(x=w437, y=16 ("length (rest)")) -> (x*y=w353:i32)
      n136 = local read "display"() -> (w420:bool)
      n137 = Add(x=w353, y=8 ("length (rest)")) -> (x+y=w410:i32)
      n138 = Add(x=w353, y=6 ("length (rest)")) -> (x+y=w387:i32)
      n139 = Add(x=w353, y=3 ("length (rest)")) -> (x+y=w357:i32)
      n140 = Add(x=w353, y=0 ("length (rest)")) -> (x+y=w396:i32)
      n141 = String Subset(string=w366, offset (0)=0, length (rest)=2 ("length (rest)")) -> (substring=w369:string)
      "name (unnamed)" <- w369
      n142 = String Subset(string=w366, offset (0)=w396, length (rest)=16 ("y")) -> (substring=w394:string)
      n143 = String Subset(string=w366, offset (0)=w396, length (rest)=8 ("length (rest)")) -> (substring=w378:string)
      "substring" <- w378
      n144 = String Subset(string=w385, offset (0)=w410, length (rest)=8 ("length (rest)")) -> (substring=w375:string)
      "substring 2" <- w375
      n145 = String Subset(string=w385, offset (0)=w387, length (rest)=6 ("length (rest)")) -> (substring=w374:string)
      "substring 3" <- w374
      n146 = Search 1D Array(1D array=w367, element=w369) -> (index of element=w370:i32)  [unwired: 1 in]
      n147 = case shown="真" w420 {
        tunnel: w434 -> [_ w473]
        frame False {
        }
        frame True {
          n148 = Index Array(array=w473, index (col)="channel for cal") -> (element=→"cal":i64[])  [unwired: 1 in]
        }
      }
      n149 = String Subset(string=w352, offset (0)=w357, length (rest)=4 ("length (rest)")) -> (substring=w355:string)
      n150 = String Length(string=w394) -> (length=w431:i32)
      n151 = Less?(x=w431, y=16) -> (x < y?=w393:bool)
      n152 = String Subset(string=w378, length (rest)=1 ("length (rest)")) -> (substring=w415:string)  [unwired: 1 in]
      n153 = String Subset(string=w378, offset (0)=7, length (rest)=1 ("length (rest)")) -> (substring=w399:string)
      n154 = Multiply(x=w370, y=w368) -> (x*y=w364:i32)
      n155 = String Subset(string=w378, offset (0)=2, length (rest)=1 ("length (rest)")) -> (substring=w376:string)
      n156 = String To Byte Array(string=w355) -> (unsigned byte array=w354:u8[])
      n157 = Equal?(x=w415, y="Z" ("format string")) -> (x = y?=w401:bool)
      n158 = Equal?(x=w399, y=w380) -> (x = y?=w400:bool)
      n159 = String To Byte Array(string=w375) -> (unsigned byte array=w407:u8[])
      n160 = String To Byte Array(string=w374) -> (unsigned byte array=w381:u8[])
      n161 = String To Byte Array(string=w376) -> (unsigned byte array=w439:u8[])
      n162 = for {
        shift-right: [w449] -> w359
        shift-left: "" ("format string") -> [w441]
        tunnel: w354 -> [w450] mode=indexing
        n163 = Number To Hexadecimal String(2:w450) -> (0:w443:string)  [unwired: 1 in]
        n164 = String Length(string=w443) -> (length=w448:i32)
        n165 = Concatenate Strings("0" ("format string"), w443) -> (w445:string)
        n166 = Equal?(x=w448, y=2) -> (x = y?=w446:bool)
        n167 = Select(t=w443, s=w446, f=w445) -> (s? t:f=w442:string)
        n168 = Concatenate Strings(w441, w442) -> (w449:string)
      }
      n169 = for {
        shift-right: [w648] -> w404
        shift-left: "" ("format string") -> [w645]
        tunnel: w439 -> [w649] mode=indexing
        n170 = Number To Hexadecimal String(2:w649) -> (0:w641:string)  [unwired: 1 in]
        n171 = String Length(string=w641) -> (length=w647:i32)
        n172 = Equal?(x=w647, y=2) -> (x = y?=w644:bool)
        n173 = Concatenate Strings("0" ("format string"), w641) -> (w643:string)
        n174 = Select(t=w641, s=w644, f=w643) -> (s? t:f=w640:string)
        n175 = Concatenate Strings(w645, w640) -> (w648:string)
      }
      n176 = for {
        shift-right: [w469] -> w405
        shift-left: "" ("format string") -> [w461]
        tunnel: w407 -> [w470] mode=indexing
        n177 = Number To Hexadecimal String(2:w470) -> (0:w463:string)  [unwired: 1 in]
        n178 = String Length(string=w463) -> (length=w468:i32)
        n179 = Concatenate Strings("0" ("format string"), w463) -> (w465:string)
        n180 = Equal?(x=w468, y=2) -> (x = y?=w466:bool)
        n181 = Select(t=w463, s=w466, f=w465) -> (s? t:f=w462:string)
        n182 = Concatenate Strings(w461, w462) -> (w469:string)
      }
      n183 = for {
        shift-right: [w459] -> w384
        shift-left: "" ("format string") -> [w451]
        tunnel: w381 -> [w460] mode=indexing
        n184 = Number To Hexadecimal String(2:w460) -> (0:w453:string)  [unwired: 1 in]
        n185 = String Length(string=w453) -> (length=w458:i32)
        n186 = Concatenate Strings("0" ("format string"), w453) -> (w455:string)
        n187 = Equal?(x=w458, y=2) -> (x = y?=w456:bool)
        n188 = Select(t=w453, s=w456, f=w455) -> (s? t:f=w452:string)
        n189 = Concatenate Strings(w451, w452) -> (w459:string)
      }
      n190 = Not(x=w393) -> (.not. x?=w392:bool)
      n191 = Compound Arithmetic op=AND(w401, w400, w392) -> (w413:bool)
      n192 = Hexadecimal String To Number(string=w404, default (0uL)=u64 0 ("default (0 U32)")) -> (number=w435:u64)  [unwired: 1 in, 1 out]
      n193 = Hexadecimal String To Number(string=w359, default (0uL)=u64 0 ("default (0 U32)")) -> (number=w350:u64)  [unwired: 1 in, 1 out]
      "trigger rate" <- w350
      n194 = Hexadecimal String To Number(string=w405, default (0uL)=u64 0 ("default (0 U32)")) -> (number=w373:u64)  [unwired: 1 in, 1 out]
      n195 = Hexadecimal String To Number(string=w384, default (0uL)=u64 0 ("default (0 U32)")) -> (number=w362:u64)  [unwired: 1 in, 1 out]
      n196 = And(x=w435, y=u64 127 ("port")) -> (x .and. y?=w365:u64)
      "channel number" <- w365
      n197 = Add(x=w364, y=w365) -> (x+y=w349:u64)
      n198 = Replace Array Subset(array=w351, new element=w350, index=w349) -> (w348:u32[])
      n199 = case shown="真" w413 {
        tunnel: w373 -> [_ w482]
        tunnel: w426 -> [w477 w497]
        tunnel: w434 -> [w480 w506]
        tunnel: [w480 w505] -> w436
        tunnel: [w479 w502] -> w432
        tunnel: w433 -> [w479 w501]
        tunnel: w349 -> [_ w487]
        tunnel: w428 -> [w478 w500]
        tunnel: [w478 w499] -> w429
        tunnel: [w477 w498] -> w427
        tunnel: w425 -> [w476 w496]
        tunnel: [w476 w495] -> w424
        tunnel: w391 -> [w475 w493]
        tunnel: [w475 w492] -> w421
        tunnel: w422 -> [_ w491]
        tunnel: w419 -> [w474 w489]
        tunnel: [w474 w488] -> w418
        tunnel: w398 -> [_ w486]
        tunnel: w397 -> [_ w485]
        tunnel: w390 -> [_ w484]
        tunnel: w362 -> [_ w483]
        tunnel: w363 -> [_ w481]
        frame False {
          (unwired) FALSE
        }
        frame True {
          n200 = Index Array(array=w496, index=w487) -> (element=w494:u32)
          n201 = Greater?(x=w494, y=w484) -> (0:w490:bool)
          n202 = And(x=w482, y=u64 1023 ("port")) -> (x .and. y?=w503:u64)
          n203 = case shown="真" w490 {
            tunnel: w506 -> [w522 w605]
            tunnel: [w521 w605] -> w505
            tunnel: w503 -> [w513 w563]
            tunnel: [w520 w595] -> w502
            tunnel: w501 -> [w520 w612]
            tunnel: w497 -> [w518 _]
            tunnel: w487 -> [w516 w593]
            tunnel: w500 -> [w519 w611]
            tunnel: [w519 w610] -> w499
            tunnel: [w518 w608] -> w498
            tunnel: w494 -> [w514 _]
            tunnel: w496 -> [w517 w607]
            tunnel: [w515 w607] -> w495
            tunnel: w494 -> [w511 _]
            tunnel: w484 -> [w508 _]
            tunnel: w493 -> [w510 w597]
            tunnel: [w509 w597] -> w492
            tunnel: w491 -> [_ w596]
            tunnel: w489 -> [w507 w590]
            tunnel: [w507 w589] -> w488
            tunnel: w487 -> [_ w586]
            tunnel: w486 -> [_ w584]
            tunnel: w485 -> [_ w585]
            tunnel: w483 -> [_ w579]
            tunnel: w483 -> [_ w568]
            tunnel: w482 -> [_ w560]
            tunnel: w481 -> [_ w558]
            frame False {
              n204 = Equal?(x=w511, y=w508) -> (x = y?=w512:bool)
              n205 = case shown="真" w512 {
                tunnel: w522 -> [w533 w539]
                tunnel: [w531 w539] -> w521
                tunnel: w517 -> [w529 w537]
                tunnel: w516 -> [w528 w534]
                tunnel: [w526 w536] -> w515
                tunnel: w514 -> [w525 w535]
                tunnel: w513 -> [w524 _]
                tunnel: w510 -> [w523 w541]
                tunnel: [w523 w540] -> w509
                frame False {
                  n206 = Index Array(array=w533, index (row)=w524, index (col)=w528) -> (element=w532:i64)
                  n207 = Increment(x=w532) -> (x+1=w530:i64)
                  n208 = Replace Array Subset(array=w533, new element=w530, index (row)=w524, index (col)=w528) -> (w531:i64[][])
                  n209 = Increment(x=w525) -> (x+1=w527:u32)
                  n210 = Replace Array Subset(array=w529, new element=w527, index=w528) -> (w526:u32[])
                  "Calibration Counter" <- w525
                }
                frame True {
                  n211 = for {
                    N: 2048 -> [_]
                    tunnel: w539 -> [w551]
                    tunnel: w534 -> [w544]
                    shift-right: [w546] -> w540
                    shift-left: w541 -> [w547]
                    i -> [w543]
                    n212 = Array Subset(array=w551, index (row)=0 ("索引"), length (row)=w543, index (col)=w544, length (col)=1 ("长度")) -> (w548:i64[][])
                    n213 = Add Array Elements(numeric array=w548) -> (sum=w545:i64)
                    n214 = Replace Array Subset(array=w547, new element=w545, index (row)=w543, index (col)=w544) -> (w546:u32[][])
                  }
                  n215 = Increment(x=w535) -> (x+1=w538:u32)
                  n216 = Replace Array Subset(array=w537, new element=w538, index=w534) -> (w536:u32[])
                }
              }
            }
            frame True {
              (unwired) 0.0 ("x")
              w602 = 0 ("索引 (行)")
              w604 = 1 ("长度")
              # "正式取数"
              n217 = And(x=w568, y=u64 31 ("port")) -> (x .and. y?=w576:u64)
              n218 = And(x=w579, y=u64 63 ("port")) -> (x .and. y?=w582:u64)
              n219 = Logical Shift(y=i16 -13, x=w582) -> (x << y=w564:u64)
              n220 = Logical Shift(y=i16 -19, x=w576) -> (x << y=w575:u64)
              n221 = And(x=w568, y=u64 63 ("port")) -> (x .and. y?=w556:u64)
              n222 = And(x=w560, y=w558) -> (x .and. y?=w559:u64)
              "fine 4" <- w559
              n223 = Multiply(x=u64 3600, y=w575) -> (x*y=w571:u64)
              n224 = Logical Shift(y=i16 -8, x=w559) -> (x << y=→"fine 3":u64)
              n225 = Multiply(x=u64 60, y=w564) -> (x*y=w572:u64)
              n226 = Logical Shift(y=i16 -10, x=w559) -> (x << y=w553:u64)
              "fine 2" <- w553
              n227 = Add(x=w572, y=w571) -> (x+y=w570:u64)
              n228 = Logical Shift(y=i16 -7, x=w556) -> (x << y=w555:u64)
              n229 = Add(x=w570, y=w555) -> (x+y=w554:u64)
              "x+y" <- w554
              n230 = Add(x=w553, y=w554) -> (x+y=w552:u64)
              n231 = Equal?(x=w586, y=u32 2) -> (x = y?=w588:bool)
              n232 = case shown="真" w588 {
                tunnel: w590 -> [w617 w620]
                tunnel: w552 -> [_ w619]
                tunnel: [w617 w618] -> w589
                frame False {
                }
                frame True {
                  n233 = Build Array (concatenate)(w620, w619) -> (w618:u64[])
                }
              }
              "cal 2" <- w589
              n234 = case shown="真" TRUE {
                tunnel: [w627 w635] -> w614
                tunnel: w605 -> [_ _]
                tunnel: w593 -> [w632 w633]
                tunnel: w563 -> [w630 w638]
                tunnel: w597 -> [w631 w639]
                frame False {
                  w626 = 0 ("index (row)")
                  w629 = 1 ("长度")
                  n235 = Decrement(x=w632) -> (x-1=w625:u64)
                  n236 = Array Subset(array=w631, index (row)=w630, length (row)=w629, index (col)=w625, length (col)=w629) -> (w628:u32[][])
                  n237 = Index Array(array=w628, index (row)=w626, index (col)=w626) -> (element=w627:u32)
                }
                frame True {
                  w634 = 0 ("index (row)")
                  w637 = 1 ("长度")
                  n238 = Array Subset(array=w639, index (row)=w638, length (row)=w637, index (col)=w633, length (col)=w637) -> (w636:u32[][])
                  n239 = Index Array(array=w636, index (row)=w634, index (col)=w634) -> (element=w635:u32)
                }
              }
              n240 = Multiply(x=w552, y=w584) -> (x*y=w567:dbl)
              n241 = Index Array(array=w611, index=w593) -> (element=w608:u32)
              n242 = Array Subset(array=w605, index (row)=w563, length (row)=w604, index (col)=w593, length (col)=w604) -> (w603:i64[][])
              n243 = Index Array(array=w603, index (row)=w602, index (col)=w602) -> (element=w601:i64)
              n244 = Divide(x=w601, y=u32 2) -> (x/y=w606:dbl)
              n245 = Increment(x=w608) -> (x+1=w609:u32)
              n246 = Add(x=w614, y=w606) -> (x+y=w613:dbl)
              n247 = Add(x=w567, y=0.0) -> (x+y=w566:dbl)
              n248 = Multiply(x=w613, y=w585) -> (x*y=w599:dbl)
              n249 = Subtract(x=w584, y=w599) -> (x-y=w583:dbl)
              n250 = Add(x=w583, y=w566) -> (x+y=w600:dbl)
              n251 = Replace Array Subset(array=w611, new element=w609, index=w593) -> (w610:u32[])
              n252 = Replace Array Subset(array=w612, new element=w600, index=w593) -> (w594:dbl[])
              n253 = case shown="真" "save data" {
                tunnel: w596 -> [_ w624]
                tunnel: w594 -> [_ w622]
                frame False {
                }
                frame True {
                  n254 = call-poly <vilib>:"Write Delimited Spreadsheet.vi"("file path (dialog if empty)"=w624, "1D data"=w622, "append to file? (new file:F)"="append csv", "delimiter (\\t)"="," ("delimiter (\\t)")) -> ()  [unwired: 10 in, 2 out]
                }
              }
              n255 = Replace Array Subset(array=w594, new element=0.0 ("new element/subarray"), index=w593) -> (w595:dbl[])
              "fine" <- w563
            }
          }
        }
      }
      n256 = Decimate 1D Array(w348) -> (→"pmt trigger rate":u32[])  [unwired: 1 out]
    }
    n257 = case shown="真" "RST" {
      tunnel: w247 -> [w344 _]
      tunnel: [w344 0] -> w270
      tunnel: [w343 w345] -> w268
      tunnel: w248 -> [w343 _]
      frame False {
      }
      frame True {
        n258 = Get Date/Time In Seconds() -> (seconds since 1Jan1904=w345:timestamp)
      }
    }
  }
  "error out 2" <- w59
  n259 = Close File(refnum=w49, error in=w81) -> (error out=→"error out":errorcluster)  [unwired: 1 out]
  n260 = call-poly <vilib>:"Write Delimited Spreadsheet.vi"("file path (dialog if empty)"=w62, "2D data"=w63, "append to file? (new file:F)"=FALSE, "transpose? (no:F)"=TRUE, "delimiter (\\t)"="," ("delimiter (\\t)")) -> ()  [unwired: 9 in, 2 out]
